vi "Co-Pilot Analyze.vi"(0 "JoystickDevRef":T1) -> (4 "Suction":bool, 6 "Ejection":bool, 8 "Auto Search?":bool, 11 "Fine Tune(RPM)":dbl, 12 "Fine Tune?":bool, 14 "Fire Override":bool, 15 "Fire":bool)   [LabVIEW 2011]
uses:
  <vilib>/Rock Robotics/WPI/Joystick/WPI_JoystickDevRef.ctl
  <vilib>/Rock Robotics/WPI/Joystick/WPI_JoystickDeviceEnum.ctl
  InfoTransferGlobal.vi
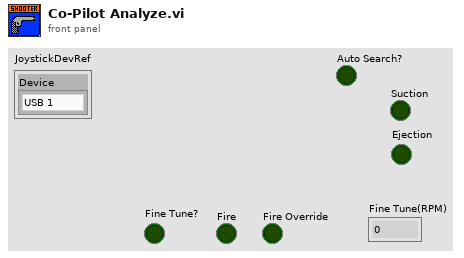
[diagram p1: front panel]
types:
  T1 = typedef "WPI_JoystickDevRef.ctl" = cluster{"Device":T2}
  T2 = typedef "WPI_JoystickDeviceEnum.ctl" = enum16{"USB 1", "USB 2", "USB 3", "USB 4", "Kinect 1", "Kinect 2"}
  T3 = cluster{"Selected Target Info":cluster{"Position":cluster{"X":dbl, "Y":dbl}, "Distance (m)":dbl, "Target Found?":bool}, "output cluster":cluster{"BottomOR":i16, "CupOR":i16, "TopOR":i16, "FloorOR":i16}, "keys pressed":enum16{"0", "1", "2", "3", "4", "5", "6", "7", "8", "9", "A", "B", "C", "D", "E", "F", "G", "H", "I", "J", "K", "L", "M", "N", "O", "P", "Q", "R", "S", "T", "U", "V", "W", "X", "Y", "Z", "F1", "F2", "F3", "F4", "F5", "F6", "F7", "F8", "F9", "F10", "F11", "F12", "F13", "F14", "F15", "ADD", "BACK", "BACKSLASH", "CAPITAL", "COMMA", "DECIMAL", "DELETE", "DIVIDE", "DOWN", "END", "EQUALS", "ESCAPE", "GRAVE (`)", "HOME", "INSERT", "LBRACKET", "LCONTROL", "LEFT", "L ALT", "LSHIFT", "LWIN", "MINUS", "MULTIPLY", "NEXT", "NUMLOCK", "NUMPAD_0", "NUMPAD_1", "NUMPAD_2", "NUMPAD_3", "NUMPAD_4", "NUMPAD_5", "NUMPAD_6", "NUMPAD_7", "NUMPAD_8", "NUMPAD_9", "PAUSE", "PERIOD", "PRIOR (PG UP)", "RBRACKET", "RCONTROL", "RETURN", "RIGHT", "R ALT", "RSHIFT", "RWIN", "SCROLL", "SEMICOLON", "SLASH", "SPACE", "SUBTRACT", "TAB", "UP", "ENTER (num pad)", "' (quote)"}[]}
  T4 = enum16{"0", "1", "2", "3", "4", "5", "6", "7", "8", "9", "A", "B", "C", "D", "E", "F", "G", "H", "I", "J", "K", "L", "M", "N", "O", "P", "Q", "R", "S", "T", "U", "V", "W", "X", "Y", "Z", "F1", "F2", "F3", "F4", "F5", "F6", "F7", "F8", "F9", "F10", "F11", "F12", "F13", "F14", "F15", "ADD", "BACK", "BACKSLASH", "CAPITAL", "COMMA", "DECIMAL", "DELETE", "DIVIDE", "DOWN", "END", "EQUALS", "ESCAPE", "GRAVE (`)", "HOME", "INSERT", "LBRACKET", "LCONTROL", "LEFT", "L ALT", "LSHIFT", "LWIN", "MINUS", "MULTIPLY", "NEXT", "NUMLOCK", "NUMPAD_0", "NUMPAD_1", "NUMPAD_2", "NUMPAD_3", "NUMPAD_4", "NUMPAD_5", "NUMPAD_6", "NUMPAD_7", "NUMPAD_8", "NUMPAD_9", "PAUSE", "PERIOD", "PRIOR (PG UP)", "RBRACKET", "RCONTROL", "RETURN", "RIGHT", "R ALT", "RSHIFT", "RWIN", "SCROLL", "SEMICOLON", "SLASH", "SPACE", "SUBTRACT", "TAB", "UP", "ENTER (num pad)", "' (quote)"}[]
  T5 = typedef "WPI_JoystickButtonState.ctl" = cluster{"Button 1":bool, "Button 2":bool, "Button 3":bool, "Button 4":bool, "Button 5":bool, "Button 6":bool, "Button 7":bool, "Button 8":bool, "Button 9":bool, "Button 10":bool, "Button 11":bool, "Button 12":bool}
  T6 = cluster{"axis 1 (x)":dbl, "axis 2 (y)":dbl, "axis 3 (throttle)":dbl, "axis 4":dbl, "axis 5":dbl, "axis 6":dbl}
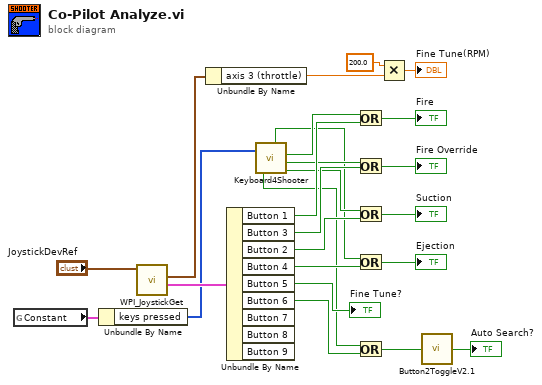
[diagram p0: block diagram]
diagram:
  n1 = global read "InfoTransferGlobal.vi" "Constant"() -> (w17:T3)
  n2 = Unbundle By Name(w17) -> ("keys pressed"=w16:T4)
  n3 = call <vilib>:"WPI_JoystickGet.vi"("JoystickDevRef"="JoystickDevRef") -> ("Buttons"=w24:T5, "Axes"=w23:T6)  [unwired: 4 in, 1 out]
  n4 = Unbundle By Name(w23) -> ("axis 3 (throttle)"=w22:dbl)
  n5 = Unbundle By Name(w24) -> ("Button 1"=w15:bool, "Button 3"=w11:bool, "Button 2"=w9:bool, "Button 4"=w6:bool, "Button 5"=→"Fine Tune?":bool, "Button 6"=w4:bool)  [unwired: 3 out]
  n6 = call "Keyboard4Shooter.vi"("1D array"=w16) -> ("Suction"=w8:bool, "ShootOR(control)"=w10:bool, "Shoot(control)"=w13:bool, "Ejection"=w5:bool, "AutoSearch"=w3:bool)  [unwired: 1 in]
  n7 = Or(x=w13, y=w15) -> (x .or. y?=→"Fire":bool)
  n8 = Or(x=w10, y=w11) -> (x .or. y?=→"Fire Override":bool)
  n9 = Or(x=w8, y=w9) -> (x .or. y?=→"Suction":bool)
  n10 = Or(x=w5, y=w6) -> (x .or. y?=→"Ejection":bool)
  n11 = Or(x=w3, y=w4) -> (x .or. y?=w2:bool)
  n12 = Multiply(x=200.0, y=w22) -> (x*y=→"Fine Tune(RPM)":dbl)
  n13 = call "Button2ToggleV2.1.vi"("a"=w2) -> ("Result(clone)"=→"Auto Search?":bool)
